vi "xml single result for8X.vi"(7 "limitType":enum16{"上限", "下限"}(ring), 8 "abs?":bool, 9 "single spec":dbl[](array[numeric]), 10 "dataSource":string[][](array[string]), 11 "second result":string) -> (2 "pointValue":string[][](array[string]), 3 "third result":string[][](array[string]))   [LabVIEW 2011]
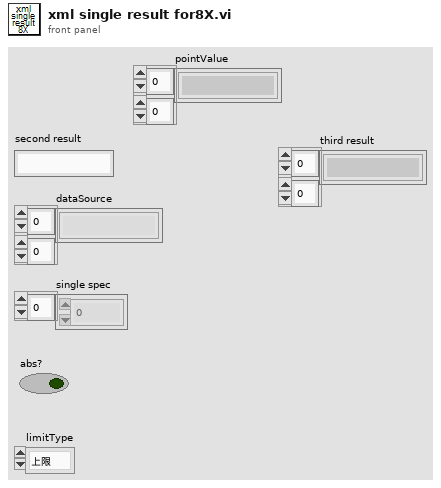
[diagram p1: front panel]
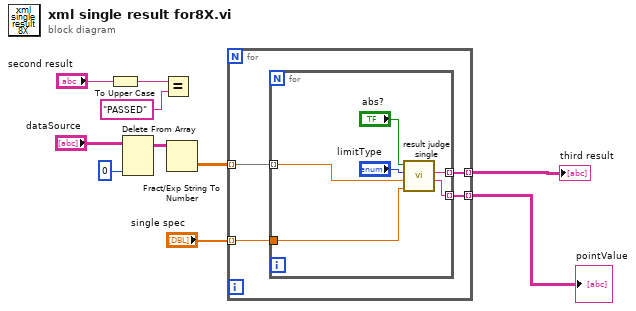
[diagram p0: block diagram]
diagram:
  n1 = To Upper Case(1:"second result") -> (0:w7:string)
  n2 = Delete From Array(array="dataSource", index (col)=0 ("禁用的索引 (列)")) -> (array with subset deleted=w3:string[][])  [unwired: 2 in, 1 out]
  n3 = Equal?(x=w7, y="PASSED") -> ()  [unwired: 1 out]
  n4 = Fract/Exp String To Number(string=w3) -> (number=w2:dbl[][])  [unwired: 3 in, 1 out]
  n5 = for {
    tunnel: w2 -> [w14] mode=indexing
    tunnel: [w13] -> w5 mode=indexing
    tunnel: "single spec" -> [w12] mode=indexing
    tunnel: [w11] -> w1 mode=indexing
    n6 = for {
      tunnel: w14 -> [w20] mode=indexing
      tunnel: [w18] -> w13 mode=indexing
      tunnel: w12 -> [w19]
      tunnel: [w15] -> w11 mode=indexing
      n7 = call "result judge single.vi"("abs?"="abs?", "limitType"="limitType", "test value"=w20, "limit"=w19) -> ("result string"=w18:string, "pointSpec"=w15:string)  [unwired: 5 in]
    }
  }
  "third result" <- w5
  "pointValue" <- w1
